vi "cw_1_2.vi"() -> ()   [LabVIEW 2022 SP3]
panel:
  in  "Starting Phase":dbl(knob) scale=0.0..360.0
  in  "Checkbox 4":bool
  in  "Checkbox 3":bool
  in  "Checkbox 2":bool
  in  "Dial":dbl(knob) scale=1.0..6.0
  in  "Checkbox":bool
  out "Measurement Progress":u8(slide) scale=0.0..100.0
  in  "Stop 4":bool
  in  "Stop 3":bool
  in  "Stop 2":bool
  in  "Start":bool
  out "Waveform Graph":dbl[](graph)
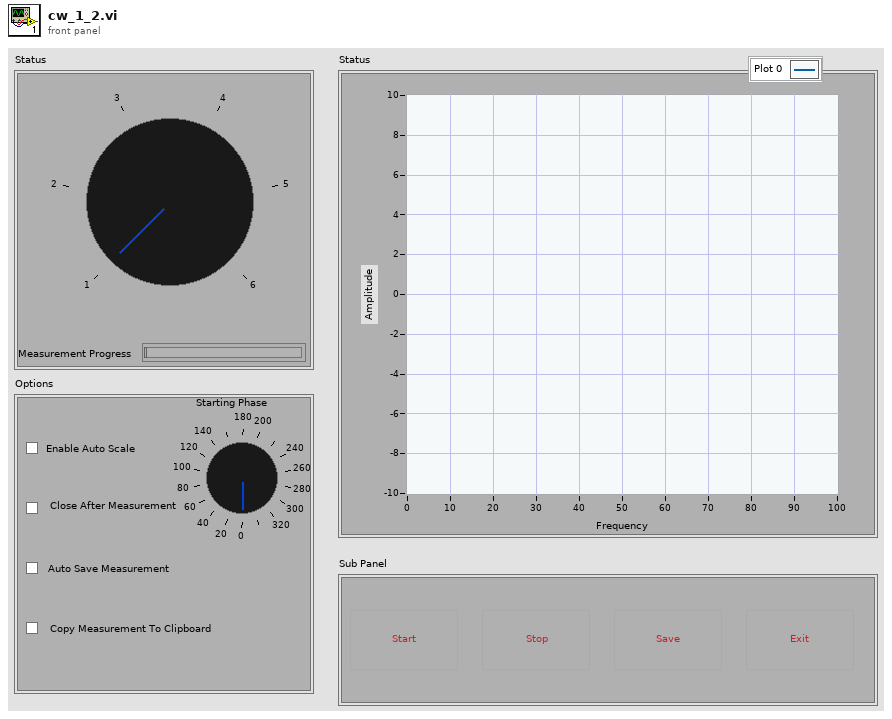
[diagram p1: front panel]
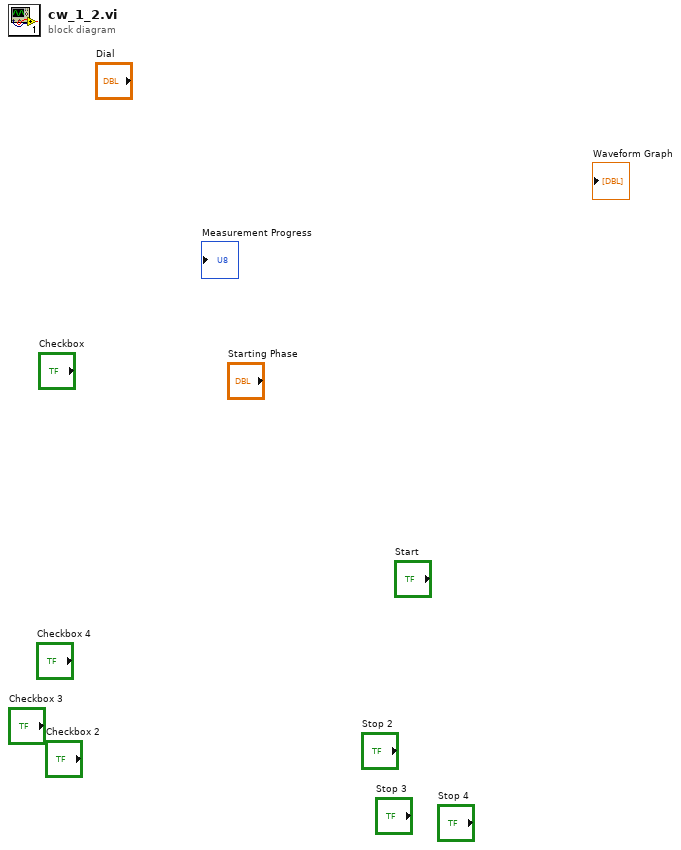
[diagram p0: block diagram]
diagram:
